vi "S_param_from_frame.VI"(0 "S-parameter Array":cdb[][](array[numeric]) format="%.2f", 5 "Frequencies (Hz)":dbl[](array[numeric]) format="%.2e", 7 "Ref Impedance":u16=75, 11 "error in (no error)":errorcluster) -> (6 "Data Output":T1={"Comments"="", "Ref Impedance"=75, "Trace Array"=[]} {"Trace Array"."Freq (Hz)" format="%.2e"; "Trace Array"."S-parameter Array" format="%.2f"}, 15 "error out":errorcluster)   [LabVIEW 2020]
doc: "Writes data in Freq S Real Imag or Magnitude Angle \n9 Column Touchstone format \nfeatures write protection for existing files"
panel:
  in  "Comments":string
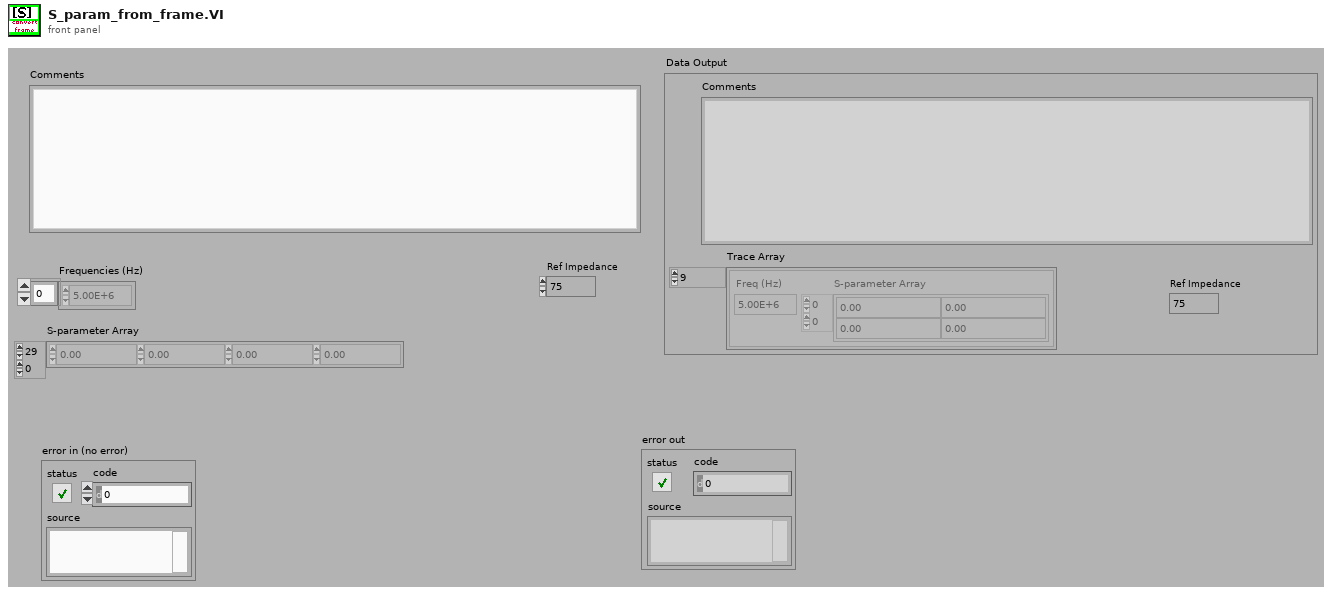
[diagram p1: front panel]
types:
  T1 = cluster{"Comments":string, "Ref Impedance":u16, "Trace Array":cluster{"Freq (Hz)":dbl, "S-parameter Array":cdb[][]}[]}
  T2 = cluster{"Freq (Hz)":dbl, "S-parameter Array":cdb[][]}[]
  T3 = cluster{"Freq (Hz)":dbl, "S-parameter Array":cdb[][]}
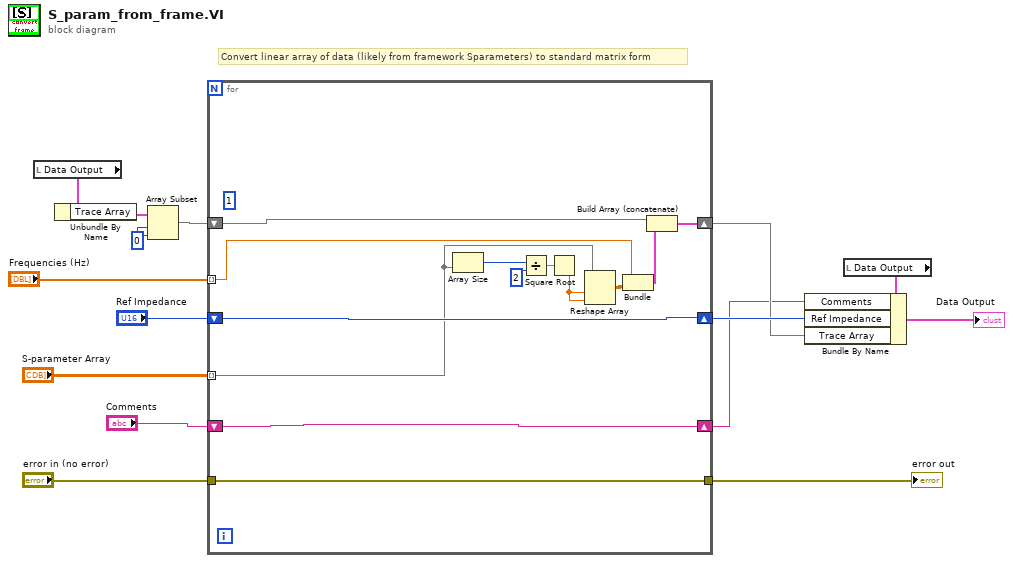
[diagram p0: block diagram]
diagram:
  w9 = 0
  # "Convert linear array of data (likely from framework Sparameters) to standard matrix form"
  n1 = local read "Data Output"() -> (w12:T1)
  n2 = Unbundle By Name(w12) -> ("Trace Array"=w11:T2)
  n3 = Array Subset(array=w11, index=w9, length=w9) -> (w10:T2)
  n4 = for {
    shift-right: [w28] -> w13
    shift-left: "Ref Impedance" -> [w28]
    shift-right: [w26] -> w8
    shift-left: w10 -> [w27]
    shift-right: [w25] -> w7
    shift-left: "Comments" -> [w25]
    tunnel: "Frequencies (Hz)" -> [w19] mode=indexing
    tunnel: "S-parameter Array" -> [w18] mode=indexing
    tunnel: [w16] -> w2
    tunnel: "error in (no error)" -> [w16]
    (unwired) 1
    n5 = Array Size(array=w18) -> (size(s)=w17:i32)
    n6 = Divide(x=w17, y=2) -> (x/y=w23:dbl)
    n7 = Square Root(x=w23) -> (sqrt(x)=w22:dbl)
    n8 = Reshape Array(w18, w22, w22) -> (w21:cdb[][])
    n9 = Bundle("Freq (Hz)"=w19, "S-parameter Array"=w21) -> (w20:T3)  [unwired: 1 out]
    n10 = Build Array (concatenate)(w27, w20) -> (w26:T2)
  }
  "error out" <- w2
  n11 = local read "Data Output"() -> (w14:T1)
  n12 = Bundle By Name(cluster=w14, "Comments"=w7, "Ref Impedance"=w13, "Trace Array"=w8) -> (→"Data Output":T1)
